vi "Test Verify JSON selects JSON Comparator.vi"(11 "Test Case In":refnum<class "Comparator Tests.lvclass">) -> (0 "error out":errorcluster, 3 "Test Case Out":refnum<class "Comparator Tests.lvclass">)   [LabVIEW 2020, in "Comparator Tests.lvclass"]
uses:
  Comparator Tests.lvclass
  C:/Program Files/National Instruments/LabVIEW 2026/vi.lib/Astemes/LUnit/Test Case.lvclass
  <vilib>/Astemes/LUnit/Test Case.lvclass/Test Case.ctl
  <vilib>/Astemes/LUnit/Core/LUnit Test Case/Private/Append Fail Result.vi
  <vilib>/Astemes/LUnit/Core/LUnit Test Case/Private/Append Pass Result.vi
  <vilib>/Astemes/LUnit/Core/LUnit Test Case/Private/Run In UI.vi
  <vilib>/Utility/error.llb/Clear Errors.vi
  <vilib>/Astemes/LUnit/Test Case.lvclass
  Source/Approval Tests/Approval Tests.lvlib
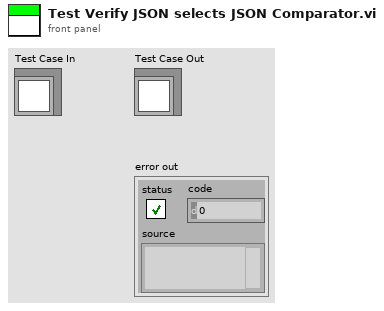
[diagram p1: front panel]
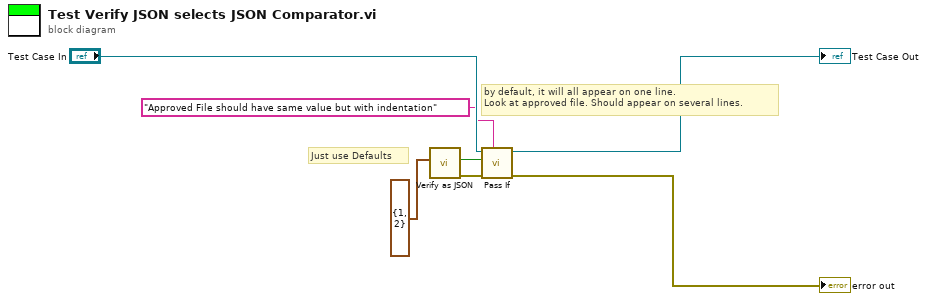
[diagram p0: block diagram]
diagram:
  # "by default, it will all appear on one line.\nLook at approved file. Should appear on several lines."
  # "Just use Defaults"
  n1 = call "Verify as JSON.vi"("Anything"=cluster{"A":i32, "B":i32} {"A"=1, "B"=2}) -> ("error out"=w6:errorcluster, "Passed?"=w3:bool)  [unwired: 8 in, 1 out]
  n2 = call <vilib>:"Pass If.vi"("Description"="Approved File should have same value but with indentation", "error in (no error)"=w6, "Pass?"=w3, "LUnit Test Case In"="Test Case In") -> ("error out"=→"error out":errorcluster, "LUnit Test Case Out"=→"Test Case Out":refnum<class "Comparator Tests.lvclass">)  [unwired: 6 in]
